vi "Editor Title.vi"(7 "Dirty (F)":bool, 10 "Entity List":refnum<vi>, 11 "VI":refnum<vi>) -> ()   [LabVIEW 2020, in "Conditum-Tools.lvlib" / "Entity Editor.lvclass"]
uses:
  Entity Editor.lvclass
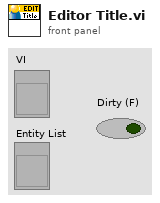
[diagram p1: front panel]
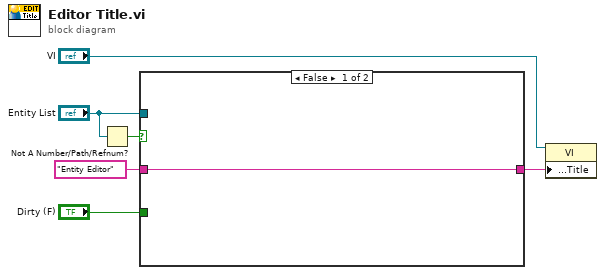
[diagram p0: block diagram]
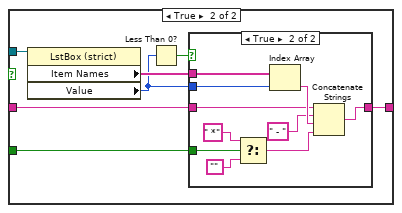
[diagram p2: hidden frame]
diagram:
  n1 = Not A Number/Path/Refnum?(number/path/refnum="Entity List") -> (NaN/Path/Refnum?=w1:bool)
  n2 = case shown="False" w1 {
    tunnel: [w7 w13] -> w6
    tunnel: "Entity List" -> [_ w12]
    tunnel: "Dirty (F)" -> [_ w11]
    tunnel: "Entity Editor" ("string") -> [w7 w10]
    frame False {
    }
    frame True {
      n3 = property on="Property Node" class="LstBox (strict)"(reference=w12) -> ("Item Names"=w14:string[], "Value"=w9:i32)  [unwired: 1 in, 2 out]
      n4 = Less Than 0?(x=w9) -> (x < 0?=w8:bool)
      n5 = case shown="True" w8 {
        tunnel: w14 -> [_ w25]
        tunnel: [w15 w23] -> w13
        tunnel: w11 -> [_ w19]
        tunnel: w10 -> [w15 w17]
        tunnel: w9 -> [_ w16]
        frame False {
        }
        frame True {
          n6 = Select(t=" *", s=w19, f="") -> (s? t:f=w18:string)
          n7 = Index Array(array=w25, index=w16) -> (element=w24:string)
          n8 = Concatenate Strings(w17, " - " ("string"), w24, w18) -> (w23:string)
        }
      }
    }
  }
  n9 = property class="VI"(reference="VI", "Front Panel.Title"=w6) -> ()  [unwired: 1 in, 2 out]
